vi "Rectangle1001.vi"   [LabVIEW 2013]
uses:
  <vilib>/Heliosphere Research LLC/Advanced Plotting Toolkit/api_core/NewPlotProperties.ctl
  <vilib>/Heliosphere Research LLC/Advanced Plotting Toolkit/typedefs/PlotColor.ctl
  <vilib>/Heliosphere Research LLC/Advanced Plotting Toolkit/api_annotations/ShapeProperties.ctl
  <vilib>/Heliosphere Research LLC/Advanced Plotting Toolkit/properties/Line.ctl
  <vilib>/Heliosphere Research LLC/Advanced Plotting Toolkit/properties/Line_Style.ctl
  <vilib>/Heliosphere Research LLC/Advanced Plotting Toolkit/properties/Display.ctl
  <vilib>/Heliosphere Research LLC/Advanced Plotting Toolkit/Advanced Plotting Toolkit.lvlib
types:
  T1 = typedef "Advanced Plotting Toolkit.lvlib/Line_Style.ctl" = enum16{"Automatic", "Solid", "Dashed", "Dotted", "Dash-dot", "Invisible"}
  T2 = typedef "Advanced Plotting Toolkit.lvlib/ShapeProperties.ctl" = cluster{"Color":T3, "Line":T4, "Display":T5}
  T3 = typedef "Advanced Plotting Toolkit.lvlib/PlotColor.ctl" = u32
  T4 = typedef "Advanced Plotting Toolkit.lvlib/Line.ctl" = cluster{"Style":T1, "Color":T3, "Width":sgl}
  T5 = typedef "Advanced Plotting Toolkit.lvlib/Display.ctl" = cluster{"Alpha":dbl, "Z Order":dbl}
  T6 = typedef "Advanced Plotting Toolkit.lvlib/NewPlotProperties.ctl" = cluster{"Background Color":T3, "Axis Background":T3, "Left Margin":dbl, "Right Margin":dbl, "Bottom Margin":dbl, "Top Margin":dbl, "Aspect Ratio":dbl}
  T7 = typedef "Advanced Plotting Toolkit.lvlib/PlotID.ctl" = i32
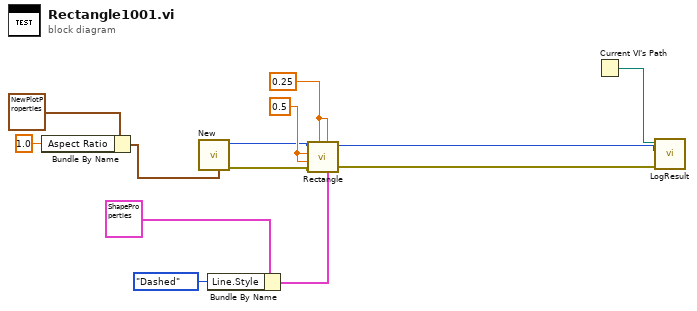
[diagram p0: block diagram]
diagram:
  w1 = 0.25 ("Radius")
  w12 = 0.5 ("X Position")
  n1 = Bundle By Name(cluster=T6 {"Background Color"=2147483647, "Axis Background"=2147483647, "Left Margin"=nan, "Right Margin"=nan, "Bottom Margin"=nan, "Top Margin"=nan, "Aspect Ratio"=nan} ("New Plot Properties"), "Aspect Ratio"=1.0) -> (w6:T6)
  n2 = call <vilib>:"New.vi"("Properties"=w6) -> ("error out"=w10:errorcluster, "Plot ID"=w11:T7)  [unwired: 9 in]
  n3 = Bundle By Name(cluster=T2 {"Color"=2147483647, "Line"={"Style"=enum."Automatic", "Color"=2147483647, "Width"=nan}, "Display"={"Alpha"=nan, "Z Order"=nan}} ("Shape Properties"), "Line.Style"=Line_Style."Dashed") -> (w3:T2)
  n4 = call <vilib>:"Rectangle.vi"("Properties"=w3, "Height"=w1, "Width"=w1, "error in (no error)"=w10, "Y Position"=w12, "X Position"=w12, "Plot ID"=w11) -> ("error out"=w8:errorcluster, "Plot ID Out"=w9:T7)  [unwired: 3 in]
  n5 = Current VI's Path() -> (path=w13:path)
  n6 = call "LogResult.vi"("Test Result"=w8, "Test Artifact"=w9, "VI Path"=w13) -> ()  [unwired: 9 in]
